vi "1762port_wvfm_builder.vi"(1 "614":digitalwaveform(waveform)={"t0"=timestamp(0 s since 1904-01-01), "dt"=0.0, "Y"={"transitions"=[], "data"=[]}, "error"={"status"=FALSE, "code"=37421928, "source"=""}}, 2 "1762":digitalwaveform(waveform)={"t0"=timestamp(0 s since 1904-01-01), "dt"=0.0, "Y"={"transitions"=[], "data"=[]}, "error"={"status"=FALSE, "code"=37421928, "source"=""}}, 3 "650":digitalwaveform(waveform)={"t0"=timestamp(0 s since 1904-01-01), "dt"=0.0, "Y"={"transitions"=[], "data"=[]}, "error"={"status"=FALSE, "code"=37421928, "source"=""}}, 4 "493":digitalwaveform(waveform)={"t0"=timestamp(0 s since 1904-01-01), "dt"=0.0, "Y"={"transitions"=[], "data"=[]}, "error"={"status"=FALSE, "code"=37421928, "source"=""}}) -> (0 "out":digitalwaveform(waveform)={"t0"=timestamp(0 s since 1904-01-01), "dt"=0.0, "Y"={"transitions"=[], "data"=[]}, "error"={"status"=FALSE, "code"=37421928, "source"=""}})   [LabVIEW 2012]
uses:
  <vilib>/Waveform/DWDTOps.llb/DWDT Append Digital Signals.vi
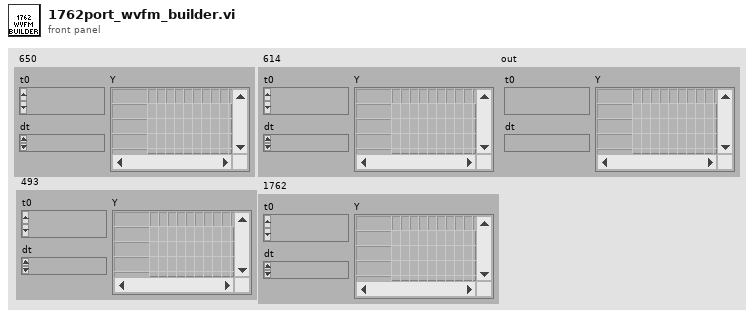
[diagram p1: front panel]
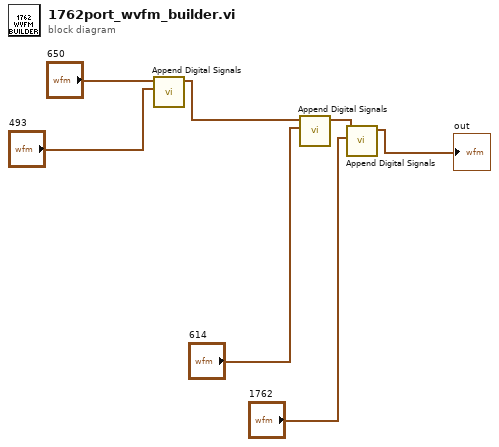
[diagram p0: block diagram]
diagram:
  n1 = call-poly <vilib>:"Append Digital Signals.vi"("digital waveform (low bits)"="493", "digital waveform (high bits)"="650") -> ("digital waveform out"=w2:digitalwaveform)  [unwired: 8 in, 1 out]
  n2 = call-poly <vilib>:"Append Digital Signals.vi"("digital waveform (low bits)"="614", "digital waveform (high bits)"=w2) -> ("digital waveform out"=w5:digitalwaveform)  [unwired: 8 in, 1 out]
  n3 = call-poly <vilib>:"Append Digital Signals.vi"("digital waveform (low bits)"="1762", "digital waveform (high bits)"=w5) -> ("digital waveform out"=→"out":digitalwaveform)  [unwired: 8 in, 1 out]
